vi "Vision Research Phantom Series PhInt PhSaturationPAR.vi"(0 "Camera Number (1)":u32=1, 3 "pPixel In":u8[](array[numeric]), 5 "Error In (no error)":errorcluster, 7 "BITMAPINFOHEADER":T5) -> (14 "Camera Number out":u32=1, 16 "pPixel":u8[](array[numeric]), 19 "Error Out":errorcluster)   [LabVIEW 2013, in "VRI.lvlib"]
doc: "PhInt.dll\n\nPhSaturationPAR\nPhSaturationPAR(int Width, int Height, int BitCount, unsigned char * pPixel, int nSaturation);\n\nParameters Description\nWidth Image width\nHeight Image height\nBitCount Bits per pixel\npPixel Pixel array pointer\nSaturation Color saturation adjustment, –100 …. +100, 0 neutral\nReturn Void\nComments A replacement for LabView of the PhSaturation function\n\nWritten by:\nBLOOMY CONTROLS, INC\nWINDSOR, CT 06095, USA\n860-298-9925\nwww.bloomy.com\nV1.0.0\nMay, 2004"
uses:
  VRI.lvlib
  _Type Defs/BITMAPINFOHEADER.ctl
  _Type Defs/PhInt WBGAIN.ctl
  _Type Defs/FilterCode.ctl
  _Type Defs/IMFILTER.ctl
  Phantom DLLs/PhInt.dll
panel:
  in  "IMPROCOPTIONS":T4 {"FilterCode" items=["PREWITT_3X3_V"=1, "PREWITT_3X3_H"=2, "SOBEL_3X3_V"=3, "SOBEL_3X3_H"=4, "LAPLACIAN_3X3"=5, "LAPLACIAN_5X5"=6, "GAUSSIAN_3X3"=7, "GAUSSIAN_5X5"=8, "HIPASS_3x3"=9, "HIPASS_5x5"=10, "SHARPEN_3X3"=11, "USERFILTER"=-1]; "Rotate" min=-90 max=90 step=1; "Saturation" min=-100 max=100 step=1; "Contrast" min=-100 max=100 step=1; "Bright" min=-100 max=100 step=1}
  # "For instructions on the use of this VI, press Ctrl+H to display the help window and move the mouse over the icon, controls, and indicators"
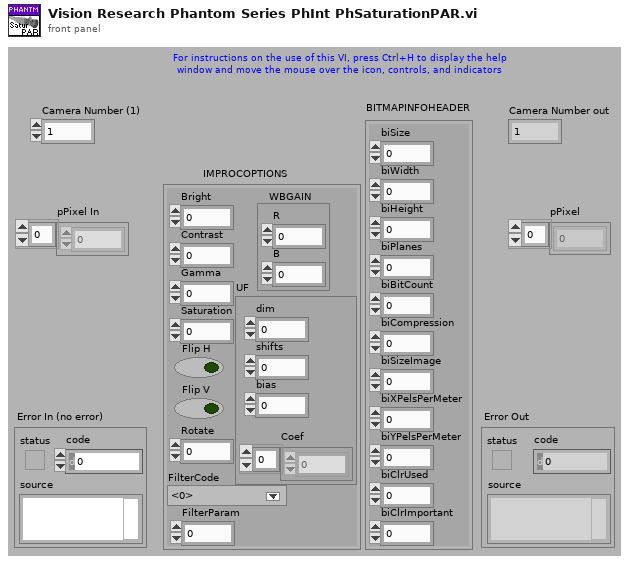
[diagram p1: front panel]
types:
  T1 = typedef "VRI.lvlib/PhInt WBGAIN.ctl" = cluster{"R":sgl, "B":sgl}
  T2 = typedef "VRI.lvlib/FilterCode.ctl" = i32
  T3 = typedef "VRI.lvlib/IMFILTER.ctl" = cluster{"dim":i32, "shifts":i32, "bias":i32, "Coef":i32[]}
  T4 = cluster{"Bright":i32, "Contrast":i32, "Gamma":sgl, "Saturation":i32, "Flip H":bool, "Flip V":bool, "Rotate":i32, "WBGAIN":T1, "FilterCode":T2, "FilterParam":i32, "UF":T3}
  T5 = typedef "VRI.lvlib/BITMAPINFOHEADER.ctl" = cluster{"biSize":u32, "biWidth":i32, "biHeight":i32, "biPlanes":u16, "biBitCount":u16, "biCompression":u32, "biSizeImage":u32, "biXPelsPerMeter":i32, "biYPelsPerMeter":i32, "biClrUsed":u32, "biClrImportant":u32}
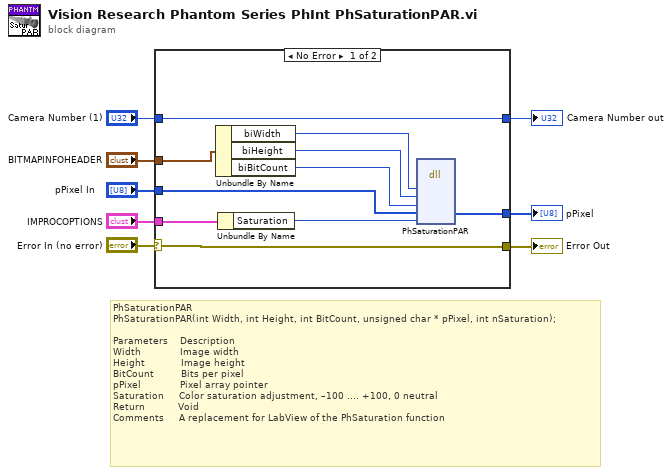
[diagram p0: block diagram]
diagram:
  # "PhSaturationPAR\nPhSaturationPAR(int Width, int Height, int BitCount, unsigned char * pPixel, int nSaturation);\n\nParameters    Description\nWidth             Image width\nHeight            Image height\nBitCount         Bits per pixel\npPixel             Pixel array pointer\nSaturation     Color saturation adjustment, –100 …. +100, 0 neutral\nReturn           Void\nComments     A replacement for LabView of the PhSaturation function"
  n1 = case shown="No Error" "Error In (no error)" {
    selector: "Error In (no error)" -> [w18 w21]
    tunnel: [w18 w21] -> w7
    tunnel: "Camera Number (1)" -> [w17 w20]
    tunnel: [w17 w20] -> w5
    tunnel: "BITMAPINFOHEADER" -> [w16 _]
    tunnel: [w15 w19] -> w3
    tunnel: "IMPROCOPTIONS" -> [w14 _]
    tunnel: "pPixel In" -> [w13 w19]
    frame No Error {
      n2 = Unbundle By Name(w16) -> ("biWidth"=w12:i32, "biHeight"=w11:i32, "biBitCount"=w10:u16)
      n3 = Unbundle By Name(w14) -> ("Saturation"=w9:i32)
      n4 = dll-call lib="C:/Projects/SDK/32-bit/Vision Research Phantom Series Labview Driver/Phantom DLLs/PhInt.dll" fn="PhSaturationPAR"("Width"=w12, "Height"=w11, "BitCount"=w10, "pPixel"=w13, "Saturation"=w9) -> ("pPixel"=w15:u8[])  [unwired: 7 in, 3 out]
    }
    frame Error {
    }
  }
  "Error Out" <- w7
  "Camera Number out" <- w5
  "pPixel" <- w3
